vi "tree_fill.vi"() -> ()   [LabVIEW 2013]
panel:
  in  "Array":string[](array[string])
  in  "Tree":string(tree)
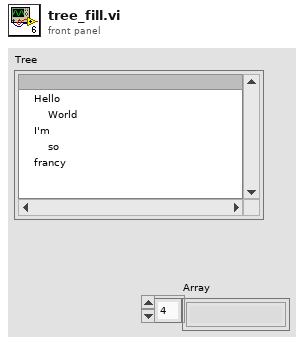
[diagram p1: front panel]
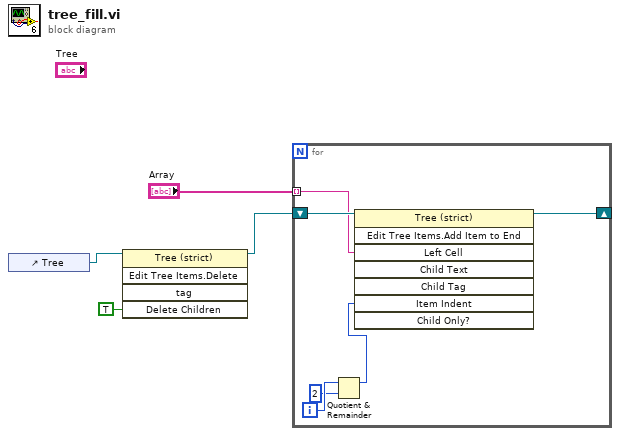
[diagram p0: block diagram]
diagram:
  n1 = control-ref of="Tree"() -> (w3:refnum<vi>)
  n2 = invoke class="Tree (strict)" method="Edit Tree Items.Delete"(reference=w3, "Delete Children"=TRUE ("Delete Children?")) -> (reference out=w2:refnum<vi>)  [unwired: 3 in, 4 out]
  n3 = for {
    shift-right: [w9] -> _
    shift-left: w2 -> [w10]
    tunnel: "Array" -> [w8] mode=indexing
    i -> [w7]
    n4 = Quotient & Remainder(x=w7, y=2) -> (x-y*floor(x/y)=w5:i32)  [unwired: 1 out]
    n5 = invoke class="Tree (strict)" method="Edit Tree Items.Add Item to End"(reference=w10, "Left Cell"=w8, "Item Indent"=w5) -> (reference out=w9:refnum<vi>)  [unwired: 5 in, 7 out]
  }
